vi "init.vi"(8 "error in (no error)":errorcluster, 9 "ILC":refnum<class "ILC.lvclass">, 10 "ILC Settings":T1={"Supply Voltage Tests"={"3.3 V Supply"={"Analog Supply DAQ Channel to Read"="AI3", "Digital Supply DAQ Channel to Read"="AI3", "Expected Value"=0.0, "Tolerance"=0.0}, "5 V Supply"={"Analog Supply DAQ Channel to Read"="AI3", "Digital Supply DAQ Channel to Read"="AI3", "Expected Value"=0.0, "Tolerance"=0.0}}, "Device Configuration Tests"={"TEDS Status Test"={"Expected Value"=""}, "Unique ID Length"=0}, "ILC Digital Input Tests"={"Limit Switch 1"={"DAQmx Global Channel"="", "High Level Value to Test"=enum."Low", "High Level Value to Expect"=enum."Low", "Low Level Value to Test"=enum."Low", "Low Level Value to Expect"=enum."Low"}, "Limit Switch 2"={"DAQmx Global Channel"="", "High Level Value to Test"=enum."Low", "High Level Value to Expect"=enum."Low", "Low Level Value to Test"=enum."Low", "Low Level Value to Expect"=enum."Low"}, "General Purpose Digital Input"={"DAQmx Global Channel"="", "High Level Value to Test"=enum."Low", "High Level Value to Expect"=enum."Low", "Low Level Value to Test"=enum."Low", "Low Level Value to Expect"=enum."Low"}}, "ILC Digital Output Tests"={"SSR"={"DAQ Channel to Read"="", "High Level Value to Test"=0, "High Level Value to Expect"=enum."Low", "Low Level Value to Test"=0, "Low Level Value to Expect"=enum."Low"}, "UART Serial Test"={"MUX Settings"={"MUX_AO"=enum."Low", "MUX_A1"=enum."Low"}, "CTS"={"DAQ Channel to Read"="", "High Level Value to Test"=0, "High Level Value to Expect"=enum."Low", "Low Level Value to Test"=0, "Low Level Value to Expect"=enum."Low"}, "TXD"={"DAQ Channel to Read"="", "High Level Value to Test"=0, "High Level Value to Expect"=enum."Low", "Low Level Value to Test"=0, "Low Level Value to Expect"=enum."Low"}, "RTS"={"DAQ Channel to Read"="", "High Level Value to Test"=0, "High Level Value to Expect"=enum."Low", "Low Level Value to Test"=0, "Low Level Value to Expect"=enum."Low"}, "RXD"={"DAQ Channel to Read"="", "High Level Value to Test"=0, "High Level Value to Expect"=enum."Low", "Low Level Value to Test"=0, "Low Level Value to Expect"=enum."Low"}}, "SSI Serial Test"={"MUX Settings"={"MUX_AO"=enum."Low", "MUX_A1"=enum."Low"}, "Out_SS"={"DAQ Channel to Read"="", "High Level Value to Test"=0, "High Level Value to Expect"=enum."Low", "Low Level Value to Test"=0, "Low Level Value to Expect"=enum."Low"}, "Out_SDI"={"DAQ Channel to Read"="", "High Level Value to Test"=0, "High Level Value to Expect"=enum."Low", "Low Level Value to Test"=0, "Low Level Value to Expect"=enum."Low"}, "Out_SCLK"={"DAQ Channel to Read"="", "High Level Value to Test"=0, "High Level Value to Expect"=enum."Low", "Low Level Value to Test"=0, "Low Level Value to Expect"=enum."Low"}, "Reset"={"DAQ Channel to Read"="", "High Level Value to Test"=0, "High Level Value to Expect"=enum."Low", "Low Level Value to Test"=0, "Low Level Value to Expect"=enum."Low"}}, "Motor Drive Test"={"MUX Settings"={"MUX_AO"=enum."Low", "MUX_A1"=enum."Low"}, "SM_CW"={"DAQ Channel to Read"="", "High Level Value to Test"=0, "High Level Value to Expect"=enum."Low", "Low Level Value to Test"=0, "Low Level Value to Expect"=enum."Low"}, "SM_CCW"={"DAQ Channel to Read"="", "High Level Value to Test"=0, "High Level Value to Expect"=enum."Low", "Low Level Value to Test"=0, "Low Level Value to Expect"=enum."Low"}, "SM_GPI"={"DAQ Channel to Read"="", "High Level Value to Expect"=enum."Low", "Low Level Value to Expect"=enum."Low", "DAQ Channel to Write"="", "High Level Value to Test"=enum."Low", "Low Level Value to Test"=enum."Low"}, "Both Free"={"LIMSW1 Level"=enum."Low", "LIMSW2 Level"=enum."Low"}, "CW Operated"={"LIMSW1 Level"=enum."Low", "LIMSW2 Level"=enum."Low"}, "CCW Operated"={"LIMSW1 Level"=enum."Low", "LIMSW2 Level"=enum."Low"}, "Both Operated"={"LIMSW1 Level"=enum."Low", "LIMSW2 Level"=enum."Low"}, "OUT_SDO"={"DAQ Channel to Read"="", "High Level Value to Test"=0, "High Level Value to Expect"=enum."Low", "Low Level Value to Test"=0, "Low Level Value to Expect"=enum."Low"}}, "MUX Signals"={"MUX_A0 DAQ Channel to Write"="", "MUX_A1 DAQ Channel to Write"=""}}, "ILC Analog Output Tests"={"Delay Between Test Steps"=0, "Vref"={"DAQ Channel to Read"="", "Expected Value"=0.0, "Tolerance"=0.0}, "ROT"={"DAQ Channel to Read"="", "Test Values"={"Start Value"=0.0, "Stop Value"=0.0, "Number of Steps"=0}, "Tolerance"=0.0}, "BIAS"={"DAQ Channel to Read"="", "Expected Value"=0.0, "Tolerance"=0.0}, "EXC"={"EXC1 DAQ Channel to Read"="", "EXC2 DAQ Channel to Read"="", "EXC3 DAQ Channel to Read"="", "EXC4 DAQ Channel to Read"="", "Expected Value"=0.0, "Tolerance"=0.0}, "DAC"={"DAC1 DAQ Channel to Read"="", "DAC2 DAQ Channel to Read"="", "DAC3 DAQ Channel to Read"="", "DAC4 DAQ Channel to Read"="", "Test Values"={"Start Value"=0.0, "Stop Value"=0.0, "Number of Steps"=0}, "Tolerance"=0.0, "Reference"=0.0}}, "ILC Analog Input Tests"={"CH13 DAQ Channel to Write"="", "CH24 DAQ Channel to Write"="", "AO Voltage Data"={"ADC Bit Count"=0, "Vref"=0.0, "NI Scaling"=0.0, "Bias"=0.0}, "Delay Between Test Steps"=0, "1 Channel"={"ADC Configurations"=[], "Value to Expect"=0, "Tolerance"=0, "PGA Gain Coefficients"=[]}, "3 Channels"={"ADC Configurations"=[], "PGA Gain Coefficients"=[], "Test Values"={"Start Value"=0.0, "Stop Value"=0.0, "Number of Steps"=0}, "Tolerance"=0.0}, "5 Channels"={"ADC Configurations"=[], "PGA Gain Coefficients"=[], "Test Values"={"Start Value"=0.0, "Stop Value"=0.0, "Number of Steps"=0}, "Tolerance"=0.0}}, "Collection Settings"={"Samples To Average"=1}, "TestExecutionOrder"=[]} {"ILC Analog Input Tests"."5 Channels"."Tolerance" format="%.9f"; "ILC Analog Input Tests"."5 Channels"."Test Values"."Stop Value" format="%.6f"; "ILC Analog Input Tests"."5 Channels"."Test Values"."Start Value" format="%.6f"; "ILC Analog Input Tests"."5 Channels"."PGA Gain Coefficients" max=7; "ILC Analog Input Tests"."3 Channels"."Tolerance" format="%.9f"; "ILC Analog Input Tests"."3 Channels"."Test Values"."Stop Value" format="%.6f"; "ILC Analog Input Tests"."3 Channels"."Test Values"."Start Value" format="%.6f"; "ILC Analog Input Tests"."3 Channels"."PGA Gain Coefficients" max=7; "ILC Analog Input Tests"."1 Channel"."PGA Gain Coefficients" max=7; "ILC Analog Input Tests"."AO Voltage Data"."Bias" min=0.0 max=10.0 format="%.3f"; "ILC Analog Input Tests"."AO Voltage Data"."NI Scaling" min=0.0 max=10.0 format="%.3f"; "ILC Analog Input Tests"."AO Voltage Data"."Vref" min=0.0 max=10.0 format="%.3f"; "ILC Analog Output Tests"."DAC"."Reference" format="%.4f"; "ILC Analog Output Tests"."DAC"."Tolerance" format="%.4f"; "ILC Analog Output Tests"."DAC"."Test Values"."Stop Value" format="%.6f"; "ILC Analog Output Tests"."DAC"."Test Values"."Start Value" format="%.6f"; "ILC Analog Output Tests"."EXC"."Tolerance" format="%.4f"; "ILC Analog Output Tests"."EXC"."Expected Value" format="%.4f"; "ILC Analog Output Tests"."BIAS"."Tolerance" format="%.4f"; "ILC Analog Output Tests"."BIAS"."Expected Value" format="%.4f"; "ILC Analog Output Tests"."ROT"."Tolerance" format="%.4f"; "ILC Analog Output Tests"."ROT"."Test Values"."Stop Value" format="%.6f"; "ILC Analog Output Tests"."ROT"."Test Values"."Start Value" format="%.6f"; "ILC Analog Output Tests"."Vref"."Tolerance" format="%.4f"; "ILC Analog Output Tests"."Vref"."Expected Value" format="%.4f"; "Supply Voltage Tests"."5 V Supply"."Tolerance" format="%.3f"; "Supply Voltage Tests"."5 V Supply"."Expected Value" format="%.3f"; "Supply Voltage Tests"."3.3 V Supply"."Tolerance" format="%.3f"; "Supply Voltage Tests"."3.3 V Supply"."Expected Value" format="%.3f"}, 11 "ITestScenarioFactory in":refnum<class "ITestScenarioFactory.lvclass">) -> (0 "error out":errorcluster, 3 "ITestScenarioFactory out":refnum<class "ITestScenarioFactory.lvclass">)   [LabVIEW 2015, in "ITestScenarioFactory.lvclass"]
uses:
  ITestScenarioFactory.lvclass
  Typedefs/ILC Settings.ctl
  Typedefs/Supply Voltage Tests.ctl
  Typedefs/Supply Voltage Test.ctl
  Typedefs/Device Configuration Tests.ctl
  Typedefs/1-Wire Test.ctl
  Typedefs/ILC Digital Input Tests.ctl
  Typedefs/ILC Digital Input Test.ctl
  Typedefs/ILC Digital Output Tests.ctl
  Typedefs/ILC Digital Output Test.ctl
  Typedefs/Digital Signal Level.ctl
  Typedefs/UART Serial Test.ctl
  Typedefs/MUX Settings.ctl
  Typedefs/SSI Serial Test.ctl
  Typedefs/Motor Drive Test.ctl
  Typedefs/ILC GPI Digital Output Test.ctl
  Typedefs/Limit Switch Configuration.ctl
  Typedefs/MUX Signals.ctl
  Typedefs/ILC Analog Output Tests.ctl
  Typedefs/ILC Static Analog Output Test.ctl
  Typedefs/ILC Analog Output Test.ctl
  Typedefs/Test Values.ctl
  Typedefs/ILC EXC Analog Output Test.ctl
  Typedefs/ILC DAC Analog Output Test.ctl
  Typedefs/ILC Analog Input Tests.ctl
  Typedefs/AI Voltage to NI Voltage.ctl
  Typedefs/ILC Ch0 Analog Input Test.ctl
  <userlib>/Common/ILC/Configuration/Scan Rates.ctl
  Typedefs/Multichannel Analog Input Test.ctl
  Typedefs/Collection Settings.ctl
  Typedefs/TestExecutionOrder.ctl
  Typedefs/TestScenarioTypes.ctl
  <userlib>/Common/ILC/ILC/ILC.lvclass
  Typedefs/ILCBTTypedefs.lvlib
  <userlib>/Common/ILC/Configuration/ILCConfiguration.lvlib
panel:
  # "AO Voltage Data"
  # "1 Channel"
  # "3 Channels"
  # "5 Channels"
  # "Vref"
  # "ROT"
  # "DAC"
  # "BIAS"
  # "EXC"
  # "Unique ID Test"
  # "TEDS Status Test"
  # "3.3 V Supply"
  # "5 V Supply"
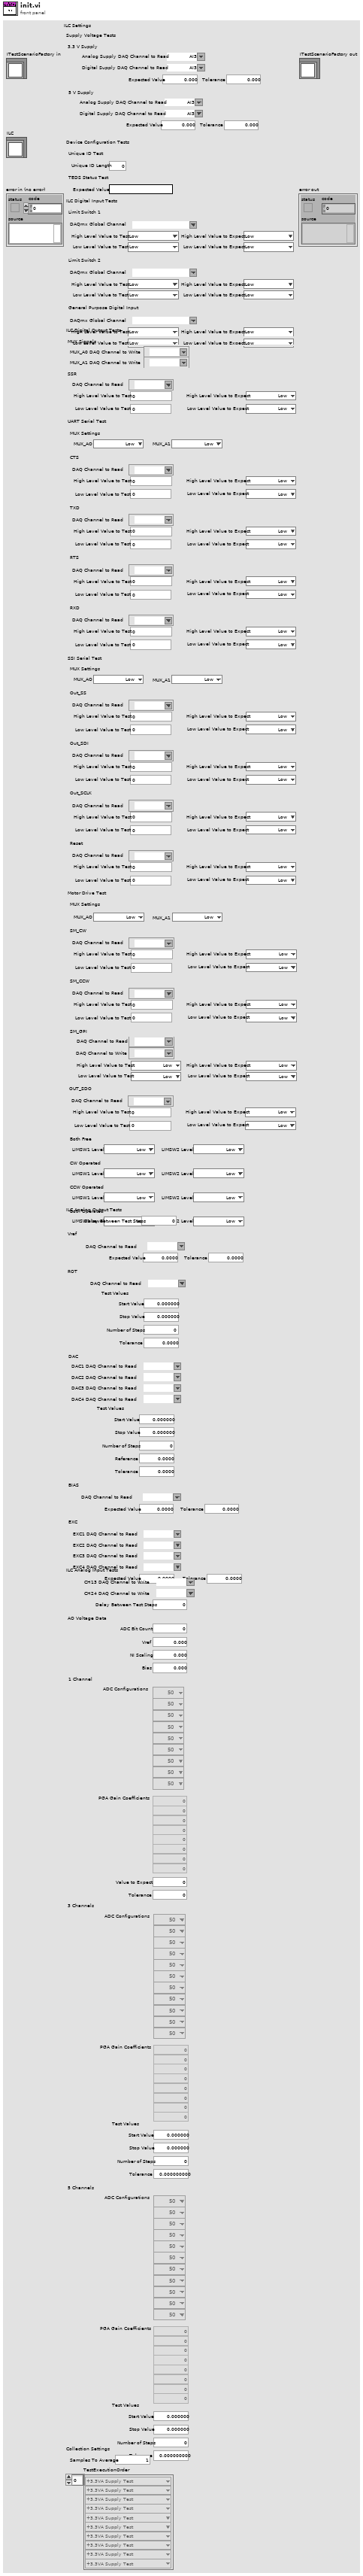
[diagram p1: front panel]
types:
  T1 = typedef "ILCBTTypedefs.lvlib/ILC Settings.ctl" = cluster{"Supply Voltage Tests":T2, "Device Configuration Tests":T4, "ILC Digital Input Tests":T6, "ILC Digital Output Tests":T8, "ILC Analog Output Tests":T18, "ILC Analog Input Tests":T24, "Collection Settings":T29, "TestExecutionOrder":T30}
  T2 = typedef "ILCBTTypedefs.lvlib/Supply Voltage Tests.ctl" = cluster{"3.3 V Supply":T3, "5 V Supply":T3}
  T3 = typedef "ILCBTTypedefs.lvlib/Supply Voltage Test.ctl" = cluster{"Analog Supply DAQ Channel to Read":refnum<k21>, "Digital Supply DAQ Channel to Read":refnum<k21>, "Expected Value":dbl, "Tolerance":dbl}
  T4 = typedef "ILCBTTypedefs.lvlib/Device Configuration Tests.ctl" = cluster{"TEDS Status Test":T5, "Unique ID Length":u8}
  T5 = typedef "ILCBTTypedefs.lvlib/1-Wire Test.ctl" = cluster{"Expected Value":string}
  T6 = typedef "ILCBTTypedefs.lvlib/ILC Digital Input Tests.ctl" = cluster{"Limit Switch 1":T7, "Limit Switch 2":T7, "General Purpose Digital Input":T7}
  T7 = typedef "ILCBTTypedefs.lvlib/ILC Digital Input Test.ctl" = cluster{"DAQmx Global Channel":refnum<k21>, "High Level Value to Test":enum16{"Low", "High"}, "High Level Value to Expect":enum16{"Low", "High"}, "Low Level Value to Test":enum16{"Low", "High"}, "Low Level Value to Expect":enum16{"Low", "High"}}
  T8 = typedef "ILCBTTypedefs.lvlib/ILC Digital Output Tests.ctl" = cluster{"SSR":T9, "UART Serial Test":T11, "SSI Serial Test":T13, "Motor Drive Test":T14, "MUX Signals":T17}
  T9 = typedef "ILCBTTypedefs.lvlib/ILC Digital Output Test.ctl" = cluster{"DAQ Channel to Read":refnum<k21>, "High Level Value to Test":u16, "High Level Value to Expect":T10, "Low Level Value to Test":u16, "Low Level Value to Expect":T10}
  T10 = typedef "ILCBTTypedefs.lvlib/Digital Signal Level.ctl" = enum16{"Low", "High"}
  T11 = typedef "ILCBTTypedefs.lvlib/UART Serial Test.ctl" = cluster{"MUX Settings":T12, "CTS":T9, "TXD":T9, "RTS":T9, "RXD":T9}
  T12 = typedef "ILCBTTypedefs.lvlib/MUX Settings.ctl" = cluster{"MUX_AO":T10, "MUX_A1":T10}
  T13 = typedef "ILCBTTypedefs.lvlib/SSI Serial Test.ctl" = cluster{"MUX Settings":T12, "Out_SS":T9, "Out_SDI":T9, "Out_SCLK":T9, "Reset":T9}
  T14 = typedef "ILCBTTypedefs.lvlib/Motor Drive Test.ctl" = cluster{"MUX Settings":T12, "SM_CW":T9, "SM_CCW":T9, "SM_GPI":T15, "Both Free":T16, "CW Operated":T16, "CCW Operated":T16, "Both Operated":T16, "OUT_SDO":T9}
  T15 = typedef "ILCBTTypedefs.lvlib/ILC GPI Digital Output Test.ctl" = cluster{"DAQ Channel to Read":refnum<k21>, "High Level Value to Expect":T10, "Low Level Value to Expect":T10, "DAQ Channel to Write":refnum<k21>, "High Level Value to Test":T10, "Low Level Value to Test":T10}
  T16 = typedef "ILCBTTypedefs.lvlib/Limit Switch Configuration.ctl" = cluster{"LIMSW1 Level":T10, "LIMSW2 Level":T10}
  T17 = typedef "ILCBTTypedefs.lvlib/MUX Signals.ctl" = cluster{"MUX_A0 DAQ Channel to Write":refnum<k21>, "MUX_A1 DAQ Channel to Write":refnum<k21>}
  T18 = typedef "ILCBTTypedefs.lvlib/ILC Analog Output Tests.ctl" = cluster{"Delay Between Test Steps":u16, "Vref":T19, "ROT":T20, "BIAS":T19, "EXC":T22, "DAC":T23}
  T19 = typedef "ILCBTTypedefs.lvlib/ILC Static Analog Output Test.ctl" = cluster{"DAQ Channel to Read":refnum<k21>, "Expected Value":dbl, "Tolerance":dbl}
  T20 = typedef "ILCBTTypedefs.lvlib/ILC Analog Output Test.ctl" = cluster{"DAQ Channel to Read":refnum<k21>, "Test Values":T21, "Tolerance":dbl}
  T21 = typedef "ILCBTTypedefs.lvlib/Test Values.ctl" = cluster{"Start Value":dbl, "Stop Value":dbl, "Number of Steps":u16}
  T22 = typedef "ILCBTTypedefs.lvlib/ILC EXC Analog Output Test.ctl" = cluster{"EXC1 DAQ Channel to Read":refnum<k21>, "EXC2 DAQ Channel to Read":refnum<k21>, "EXC3 DAQ Channel to Read":refnum<k21>, "EXC4 DAQ Channel to Read":refnum<k21>, "Expected Value":dbl, "Tolerance":dbl}
  T23 = typedef "ILCBTTypedefs.lvlib/ILC DAC Analog Output Test.ctl" = cluster{"DAC1 DAQ Channel to Read":refnum<k21>, "DAC2 DAQ Channel to Read":refnum<k21>, "DAC3 DAQ Channel to Read":refnum<k21>, "DAC4 DAQ Channel to Read":refnum<k21>, "Test Values":T21, "Tolerance":dbl, "Reference":dbl}
  T24 = typedef "ILCBTTypedefs.lvlib/ILC Analog Input Tests.ctl" = cluster{"CH13 DAQ Channel to Write":refnum<k21>, "CH24 DAQ Channel to Write":refnum<k21>, "AO Voltage Data":T25, "Delay Between Test Steps":u16, "1 Channel":T26, "3 Channels":T28, "5 Channels":T28}
  T25 = typedef "ILCBTTypedefs.lvlib/AI Voltage to NI Voltage.ctl" = cluster{"ADC Bit Count":u16, "Vref":dbl, "NI Scaling":dbl, "Bias":dbl}
  T26 = typedef "ILCBTTypedefs.lvlib/ILC Ch0 Analog Input Test.ctl" = cluster{"ADC Configurations":T27[], "Value to Expect":i32, "Tolerance":i32, "PGA Gain Coefficients":u16[]}
  T27 = typedef "ILCCommon.lvlib/ILCConfiguration.lvlib/Scan Rates.ctl" = enum16{"50", "60", "100", "120", "200", "240", "300", "400", "480", "600", "1200", "2400", "4800"}
  T28 = typedef "ILCBTTypedefs.lvlib/Multichannel Analog Input Test.ctl" = cluster{"ADC Configurations":T27[], "PGA Gain Coefficients":u16[], "Test Values":T21, "Tolerance":dbl}
  T29 = typedef "ILCBTTypedefs.lvlib/Collection Settings.ctl" = cluster{"Samples To Average":i32}
  T30 = typedef "ILCBTTypedefs.lvlib/TestExecutionOrder.ctl" = T31[]
  T31 = typedef "ILCBTTypedefs.lvlib/TestScenarioTypes.ctl" = enum16{"+3.3VA Supply Test", "+3.3VD Supply Test", "+5VA Supply Test", "+5VD Supply Test", "Unique ID Test", "TEDS Status Test", "LIMSW1_TTL Low Test", "LIMSW1_TTL High Test", "LIMSW2_TTL Low Test", "LIMSW2_TTL High Test", "Tachometer Low Test", "Tachometer High Test", "SSR_TTL Low Test", "SSR_TTL High Test", "SM_GPI Low Test", "SM_GPI High Test", "CW Motion Without Limit Test", "CW Motion With Limit Test", "CW Motion With Both Limits Test", "CW Motion on CCW Limit Test", "CCW Motion Without Limit Test", "CCW Motion With Limit Test", "CCW Motion With Both Limits Test", "CCW Motion on CW Limit Test", "OUT_SDO Low Test", "OUT_SDO High Test", "RS232-TXD Low Test", "RS232-TXD High Test", "RS232-RTS Low Test", "RS232-RTS High Test", "RS232-RXD Low Test", "RS232-RXD High Test", "RS232-CTS Low Test", "RS232-CTS High Test", "Out_SS Low Test", "Out_SS High Test", "Out_SDI Low Test", "Out_SDI High Test", "Out_SCLK Low Test", "Out_SCLK High Test", "Reset Low Test", "Reset High Test", "1 Channel ADC Test", "3 Channel ADC Test", "5 Channel ADC Test", "Vref Test", "ROT Test", "DAC1 Test", "DAC2 Test", "DAC3 Test", "DAC4 Test", "BIAS Test", "EXC1 Test", "EXC2 Test", "EXC3 Test", "EXC4 Test"}
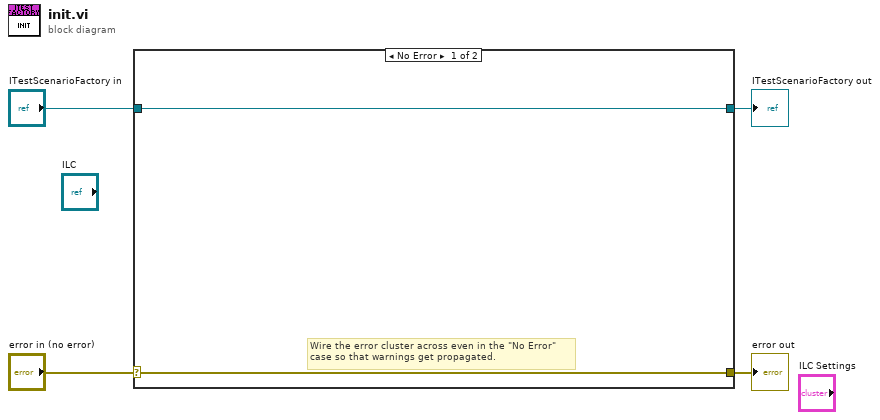
[diagram p0: block diagram]
diagram:
  n1 = case shown="No Error" "error in (no error)" {
    selector: "error in (no error)" -> [w5 w8]
    tunnel: [w5 w8] -> w3
    tunnel: [w6 w7] -> w1
    tunnel: "ITestScenarioFactory in" -> [w6 w7]
    frame No Error {
      # "Wire the error cluster across even in the \"No Error\"\ncase so that warnings get propagated."
    }
    frame Error {
    }
  }
  "error out" <- w3
  "ITestScenarioFactory out" <- w1
